vi "Actor Core.vi"(8 "error in":errorcluster, 11 "Simulated Screen Interface in":refnum<class "Simulated Screen Interface.lvclass">) -> (0 "error out":errorcluster, 3 "Actor out":refnum<class "Actor.lvclass">)   [LabVIEW 2017, in "Simulated Screen Interface.lvlib" / "Simulated Screen Interface.lvclass"]
doc: "(<B>Filename</B>: Actor Framework.lvlib:Actor.lvclass:Actor Core.vi)\n\nReceives messages to the actor, reacts to them, and initiates any error handling that may shut the actor down.\n\nDescendant classes may override this VI to append parallel tasks for the actor to complete while it handles messages. Overrides use the Call Parent Method node."
uses:
  Simulated Screen Interface.lvclass
  <vilib>/ActorFramework/Actor/Actor.lvclass
  Screen Interface/Screen Interface/Screen Interface.lvclass
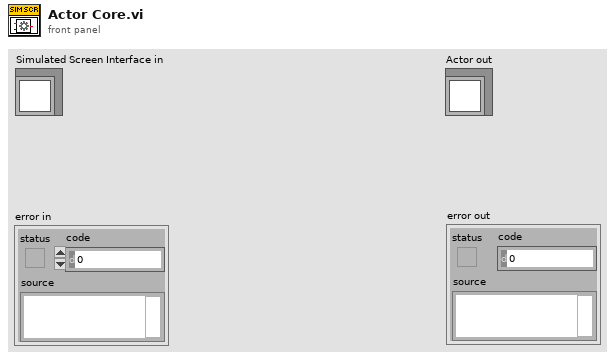
[diagram p1: front panel]
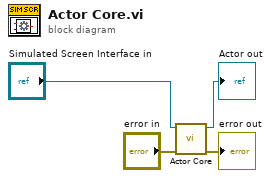
[diagram p0: block diagram]
diagram:
  n1 = call-parent "Actor Core.vi"("error in"="error in", "Screen Interface in"="Simulated Screen Interface in") -> ("error out"=→"error out":errorcluster, "Actor out"=→"Actor out":refnum<class "Actor.lvclass">)  [unwired: 8 in]
